vi "Update Table Value & Format.vi"(8 "error in (no error)":errorcluster, 11 "Protocol Verification Test in":refnum<class "Protocol Verification Test.lvclass">) -> (0 "error out":errorcluster, 3 "Protocol Verification Test out":refnum<class "Protocol Verification Test.lvclass">)   [LabVIEW 2017, in "Protocol Verification Test.lvlib" / "Protocol Verification Test.lvclass"]
uses:
  Protocol Verification Test.lvclass
  <vilib>/Utility/miscctls.llb/LVRowAndColumnTypeDef.ctl
  Protocol Verification Test.lvclass/Protocol Verification Test.ctl
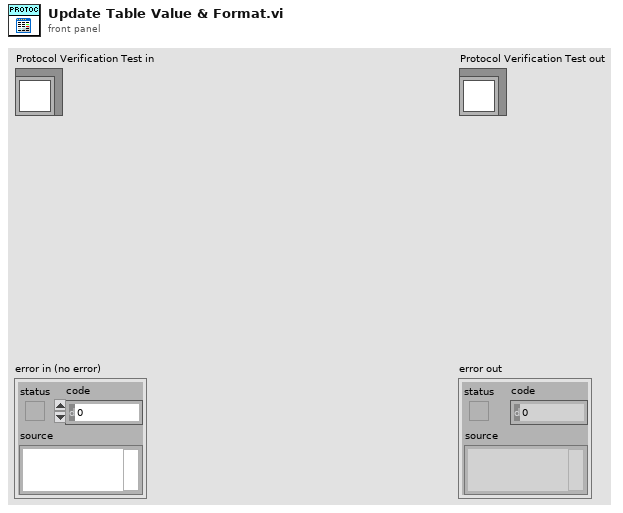
[diagram p1: front panel]
types:
  T1 = typedef "LVRowAndColumnTypeDef.ctl" = cluster{"Row":i32, "Column":i32}
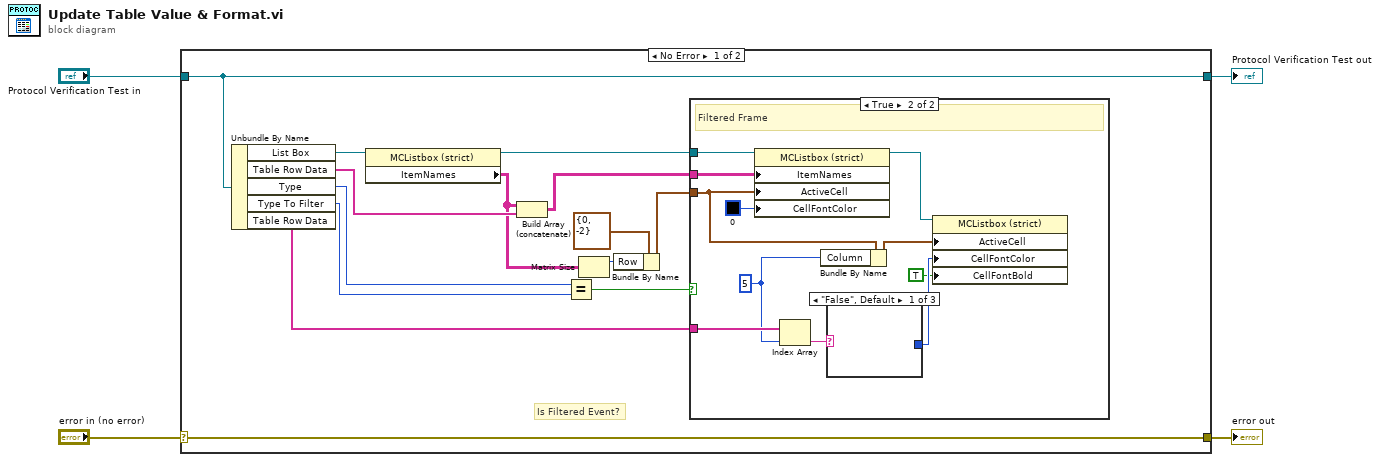
[diagram p0: block diagram]
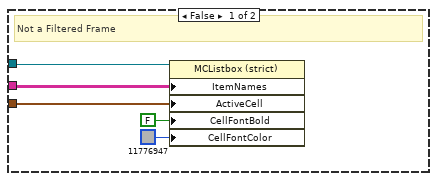
[diagram p2: hidden frame]
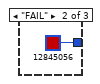
[diagram p3: hidden frame]
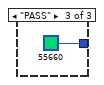
[diagram p4: hidden frame]
diagram:
  n1 = case shown="No Error" "error in (no error)" {
    selector: "error in (no error)" -> [w18 w38]
    tunnel: [w18 w38] -> w3
    tunnel: [w17 w37] -> w1
    tunnel: "Protocol Verification Test in" -> [w17 w37]
    frame No Error {
      # "Is Filtered Event?"
      n2 = Unbundle By Name(w17) -> ("List Box"=w16:refnum<vi>, "Table Row Data"=w14:string[], "Type"=w9:u8, "Type To Filter"=w8:i32, "Table Row Data"=w6:string[])
      n3 = property class="MCListbox (strict)"(reference=w16) -> (reference out=w15:refnum<vi>, "ItemNames"=w5:string[][])  [unwired: 1 in, 1 out]
      n4 = Build Array (concatenate)(w5, w14) -> (w10:string[][])
      n5 = Equal?(x=w9, y=w8) -> (x = y?=w7:bool)
      n6 = Matrix Size(0:w5) -> (1:w11:i32)  [unwired: 1 out]
      n7 = Bundle By Name(cluster=T1 {"Row"=0, "Column"=-2} ("Active Cell:Active Cell"), "Row"=w11) -> (w12:T1)
      n8 = case shown="True" w7 {
        tunnel: w15 -> [w21 w34]
        tunnel: w12 -> [w19 w30]
        tunnel: w10 -> [w20 w33]
        tunnel: w6 -> [_ w28]
        frame False {
          # "Not a Filtered Frame"
          n9 = property class="MCListbox (strict)"(reference=w21, "ItemNames"=w20, "ActiveCell"=w19, "CellFontBold"=FALSE ("Active Cell:Cell Font:Bold"), "CellFontColor"=u32 11776947 ("Color Box")) -> ()  [unwired: 1 in, 2 out]
        }
        frame True {
          w25 = 5 ("index")
          # "Filtered Frame"
          n10 = property class="MCListbox (strict)"(reference=w34, "ItemNames"=w33, "ActiveCell"=w30, "CellFontColor"=u32 0 ("Color Box")) -> (reference out=w31:refnum<vi>)  [unwired: 1 in, 1 out]
          n11 = Index Array(array=w28, index=w25) -> (element=w27:string)
          n12 = Bundle By Name(cluster=w30, "Column"=w25) -> (w29:T1)
          n13 = case shown="\"False\", Default" w27 {
            tunnel: [_ u32 12845056 ("Color Box") u32 55660 ("Color Box")] -> w26
            frame "False", Default {
            }
            frame "FAIL" {
            }
            frame "PASS" {
            }
          }
          n14 = property class="MCListbox (strict)"(reference=w31, "ActiveCell"=w29, "CellFontColor"=w26, "CellFontBold"=TRUE ("Active Cell:Cell Font:Bold")) -> ()  [unwired: 1 in, 2 out]
        }
      }
    }
    frame Error {
    }
  }
  "error out" <- w3
  "Protocol Verification Test out" <- w1
